vi "Get_Spec_Frequency.vi"(8 "error in (no error)":errorcluster, 11 ".NET Reference in":refnum<k24>) -> (0 "error out":errorcluster, 1 "minfreq":dbl, 2 "maxfreq":dbl, 3 "Reference out":refnum<k24>)   [LabVIEW 2017]
uses:
  D:/test/FULLband-sts/Fullband_Sample/DLL/InstrumentDLL.dll
  DLL/InstrumentDLL.dll
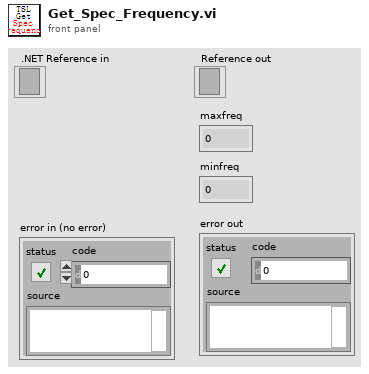
[diagram p1: front panel]
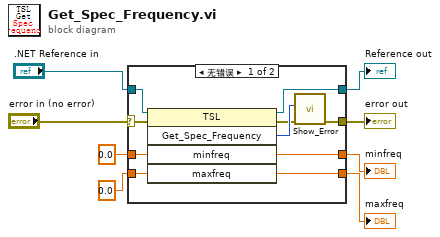
[diagram p0: block diagram]
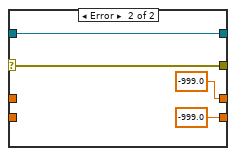
[diagram p2: hidden frame]
diagram:
  n1 = case shown="无错误" "error in (no error)" {
    selector: "error in (no error)" -> [w9 w22]
    tunnel: ".NET Reference in" -> [w18 w21]
    tunnel: [w17 w21] -> w7
    tunnel: [w10 w22] -> w6
    tunnel: 0.0 ("minwave") -> [w16 _]
    tunnel: 0.0 ("maxwave") -> [w15 _]
    tunnel: [w14 -999.0 ("minfreq")] -> w3
    tunnel: [w13 -999.0 ("maxfreq")] -> w2
    frame No Error {
      n2 = invoke on="调用节点" class="TSL" method="Get_Spec_Frequency"(reference=w18, error in=w9, "minfreq"=w16, "maxfreq"=w15) -> (reference out=w17:refnum<k24>, error out=w11:errorcluster, "Get_Spec_Frequency"=w12:i32, "minfreq"=w14:dbl, "maxfreq"=w13:dbl)  [unwired: 1 in]
      n3 = call "Show_Error.vi"("error in (no error)"=w11, "Error"=w12) -> ("error out"=w10:errorcluster)  [unwired: 9 in]
    }
    frame Error {
    }
  }
  "Reference out" <- w7
  "error out" <- w6
  "minfreq" <- w3
  "maxfreq" <- w2
